vi "Investigate Charge States.vi"() -> ()   [LabVIEW 2010]
uses:
  Drivers/Telemetry/Typedef Command List.ctl
  <instrlib>/Agilent 33XXX Series/Agilent 33XXX Series.lvlib
panel:
  out "XY Graph":cluster{"Y":dbl[], "Y":dbl[]}[](graph)
  out "Array 2":u32[](array[numeric])
  out "Array":string[](array[string])
  in  "stop":bool
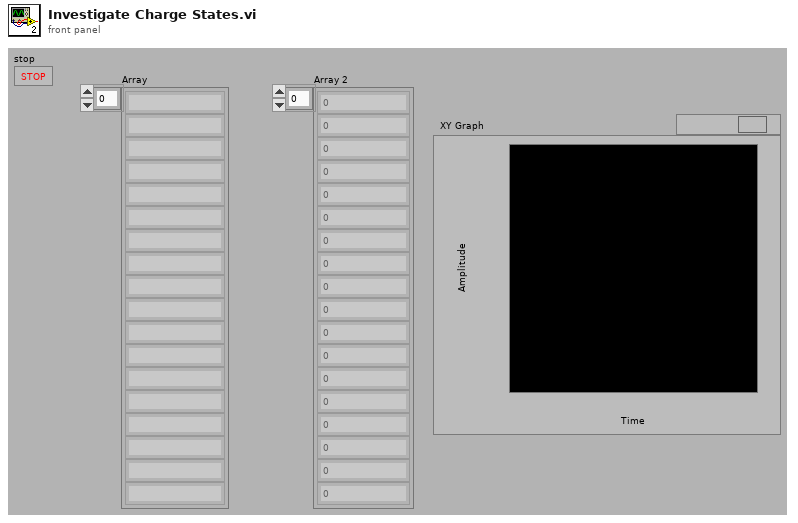
[diagram p1: front panel]
types:
  T1 = enum16{"Open Session", "Close Session", "Downlink Only", "Uplink Only", "Transceive (DN -> UP)"}
  T2 = typedef "Typedef Command List.ctl" = enum16{"Get xPG Status", "xPG Stimulation", "Select Program", "Increment Program Amplitude", "Decrement Program Amplitude", "Get PoP Constants", "Get PPC Constants", "Get Program Names", "Set Pulse Amplitude", "Increment Pulse Amplitude", "Decrement Pulse Amplitude", "Get Pulse Widths", "Set Pulse Widths", "Increment Pulse Width", "Decrement Pulse Width", "Get Program Frequency", "Set Program Frequency", "Increment Program Frequency", "Decrement Program Frequency", "Inject Event", "Charging Control", "Get xPG Identity", "Set xPG Identity", "Restore Program Defaults", "Get Program Definition", "Set Program Definition", "Get Program Constants", "Set Program Constants", "Get Configurable Device Parameters", "Set Configurable Device Parameters", "Get Pulse Constants", "Set Pulse Constants", "Get Lead Limits", "Set Lead Limits", "Get Channel Calibrations", "Set Channel Calibrations", "<reserved 2>", "<reserved 3>", "<reserved 4>", "<reserved 5>", "<reserved 6>", "<reserved 7>", "Get Stim Asic HV Calibrations", "Set Stim Asic HV Calibrations", "<reserved 8>", "<reserved 9>", "Get CP Data", "Set CP Data", "Clear Log", "Read Log", "Append Log", "Get Patient Program Runtime", "Set Patient Program Runtime", "Impedance Measurement", "Enter Storage Mode", "Echo Short", "Echo Long", "Get General Calibration", "Set General Calibration", "Get Trim List", "Set Trim List", "Get Counter", "Set Counter", "Get Test Stimulation", "Set Test Stimulation", "Get Titration Stimulation", "Set Titration Stimulation", "Get Ramp Time", "Set Ramp Time", "Get VBAT", "Set Software Description Block", "Get Software Description Block", "Write Memory", "Read Memory", "Reset xPG", "Erase Flash Block", "Write Vectors", "Read Vectors", "Diagnostic Data", "Set Background Impedance", "Get Background Impedence ", "Undefined"}
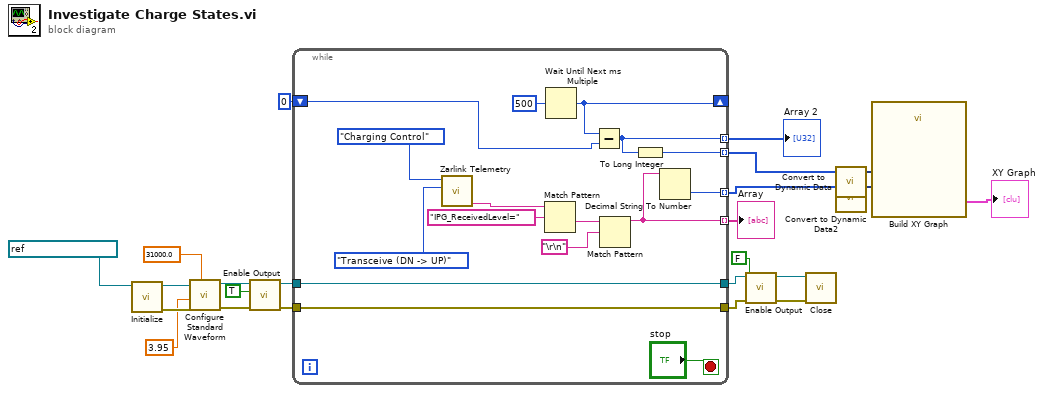
[diagram p0: block diagram]
diagram:
  n1 = call <instrlib>:"Initialize.vi"("VISA resource name"=refnum<visa-resource-name> "GPIB0::7::INSTR") -> ("error out"=w20:errorcluster, "VISA resource name out"=w19:refnum<visa-resource-name>)  [unwired: 9 in]
  n2 = call <instrlib>:"Configure Standard Waveform.vi"("Frequency (1000 Hz)"=31000.0, "error in (no error)"=w20, "Amplitude (1)"=3.95, "VISA resource name"=w19) -> ("error out"=w18:errorcluster, "VISA resource name out"=w17:refnum<visa-resource-name>)  [unwired: 6 in]
  n3 = call <instrlib>:"Enable Output.vi"("error in (no error)"=w18, "Enable Output  (T: Enable)"=TRUE, "VISA resource name"=w17) -> ("error out"=w13:errorcluster, "VISA resource name out"=w16:refnum<visa-resource-name>)  [unwired: 7 in]
  n4 = while {
    tunnel: [w27] -> w22 mode=indexing
    shift-right: [w28] -> _
    shift-left: u32 0 ("millisecond timer value") -> [w29]
    tunnel: [w26] -> w21 mode=indexing
    tunnel: w16 -> [w32]
    tunnel: [w32] -> w15
    tunnel: w13 -> [w31]
    tunnel: [w31] -> w12
    tunnel: [w25] -> w2 mode=indexing
    tunnel: [w24] -> w4 mode=indexing
    stop <- "stop" stop-if-true
    n5 = call "Zarlink Telemetry.vi"("Function"=T1."Transceive (DN -> UP)", "Command"=Typedef_Command_List."Charging Control") -> ("Data"=w38:string)  [unwired: 4 in, 5 out]
    n6 = Match Pattern(string=w38, regular expression="IPG_ReceivedLevel=") -> (after substring=w36:string)  [unwired: 1 in, 3 out]
    n7 = Wait Until Next ms Multiple(millisecond multiple=u32 500) -> (millisecond timer value=w28:u32)
    n8 = Subtract(x=w28, y=w29) -> (x-y=w26:u32)
    n9 = Match Pattern(string=w36, regular expression="\r\n") -> (before substring=w27:string)  [unwired: 1 in, 3 out]
    n10 = To Long Integer(number=w26) -> (32bit integer=w24:i32)
    n11 = Decimal String To Number(string=w27) -> (number=w25:i32)  [unwired: 2 in, 1 out]
  }
  "Array" <- w22
  "Array 2" <- w21
  n12 = call <instrlib>:"Enable Output.vi"("error in (no error)"=w12, "Enable Output  (T: Enable)"=FALSE, "VISA resource name"=w15) -> ("error out"=w11:errorcluster, "VISA resource name out"=w14:refnum<visa-resource-name>)  [unwired: 7 in]
  n13 = call <instrlib>:"Close.vi"("error in (no error)"=w11, "VISA resource name"=w14) -> ()  [unwired: 9 in, 1 out]
  n14 = call "Convert to Dynamic Data"("Array"=w4) -> ("Dynamic Data Type"=w3:dynamicdata)  [unwired: 3 in]
  n15 = call "Convert to Dynamic Data2"("Array"=w2) -> ("Dynamic Data Type"=w1:dynamicdata)  [unwired: 3 in]
  n16 = call "Build XY Graph"("Y Input"=w1, "X Input"=w3) -> ("XY Graph"=→"XY Graph":cluster{"Y":dbl[], "Y":dbl[]}[])  [unwired: 3 in, 6 out]
